vi "TriggerInput.vi"(9 "Ok to read":bool, 10 "Continous":bool, 11 "Trigger input":bool) -> (3 "out":bool)   [LabVIEW 2013]
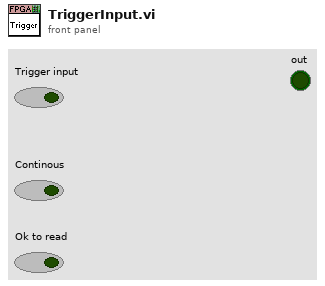
[diagram p1: front panel]
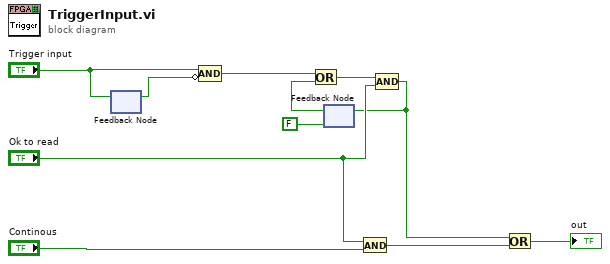
[diagram p0: block diagram]
diagram:
  n1 = feedback #1() -> (w6:bool)  [unwired: 1 in]
  n2 = feedback-in #1("Trigger input") -> ()
  n3 = Compound Arithmetic op=AND("Trigger input", invert w6) -> (w4:bool)
  n4 = feedback #2(FALSE) -> (w7:bool)
  n5 = Or(x=w4, y=w7) -> (x .or. y?=w9:bool)
  n6 = And(x="Ok to read", y="Continous") -> (x .and. y?=w10:bool)
  n7 = Compound Arithmetic op=AND(w9, "Ok to read") -> (w2:bool)
  n8 = feedback-in #2(w2) -> ()
  n9 = Or(x=w2, y=w10) -> (x .or. y?=→"out":bool)
